vi "DHT11 Read (FPGA).vi"(0 "FPGA I/O In":refnum<k21>="ConnectorA/DIO0") -> (4 "Temperature (°C)":u8, 6 "Humidity (%)":u8, 15 "error out":errorcluster)   [LabVIEW 2015, in "DHT11 (FPGA).lvlib"]
doc: "Read Temperature and Humidity from DHT11 Sensor.\n\n\nError Codes\n========\n\nError -8001: Checksum Error\nError- 8002: Timeout Error"
uses:
  DHT11 (FPGA).lvlib
  Command.ctl
  <vilib>/Platform/TimedLoop/XDataNode/timing_clust.ctl
  <vilib>/Platform/TimedLoop/XDataNode/nitl_modes.ctl
  <vilib>/Platform/TimedLoop/XDataNode/wakeup.ctl
  <vilib>/rvi/Emulation/niFpgaSctlEmulationGetInTimedLoop.vi
  <vilib>/rvi/Emulation/niFpgaEmulationReportErrorSimple.vi
  <vilib>/rvi/Emulation/niFpgaGetClockAttributes.vi
  <vilib>/rvi/Emulation/niFpgaCriticalErrorInLSC.vi
  <vilib>/rvi/eio/common/nirviEmuTemplateMethod_errors.vi
  <vilib>/Platform/TimedLoop/XDataNode/XDataNode.xnode
  <vilib>/eio/EIOMethodNode/EIOMethodNode.xnode
  <vilib>/eio/EIONode/EIONode.xnode
  <vilib>/Platform/TimedLoop/XDataNode/XDNodeRunTimeDep.lvlib
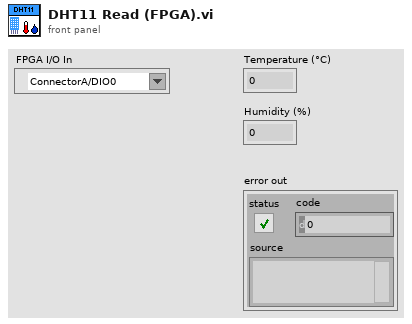
[diagram p1: front panel]
types:
  T1 = typedef "DHT11 (FPGA).lvlib/Command.ctl" = enum16{"Send Start Signal", "Wait Low", "Host Pulls Up", "Wait High", "Change to Read", "Wait for Sensor Response Signal Low", "Wait for Sensor Response Signal High", "Start Data Transmission", "Read Data", "Scale and Checksum", "Checksum Error", "Timeout Error"}
  T2 = typedef "XDNodeRunTimeDep.lvlib/timing_clust.ctl" = cluster{"Expected End [f-1]":u64, "Actual End [f-1]":u64, "Finished Late? [f-1]":bool, "Expected End [i-1]":u64, "Actual End [i-1]":u64, "Finished Late? [i-1]":bool, "Expected Start [i]":u64, "Actual Start [i]":u64, "Expected Start [f]":u64, "Actual Start [f]":u64, "Source Name":string, "Structure Name":string, "Period":i64, "Deadline":i64, "Offset":i64, "Start":i64, "Priority":i32, "Timeout":i32, "Mode":T3, "Wakeup Reason":T4, "Error":errorcluster, "Source Type":string, "Secondary Source Type":string, "Global End Time":u64, "Global Start Time":u64, "Frame Duration":u64, "Iteration Duration":u64, "Assigned CPU":i32, "I/O Scan Engine Mode":u32}
  T3 = typedef "XDNodeRunTimeDep.lvlib/nitl_modes.ctl" = enum32{"No Change", "Process missed periods, maintain original phase", "Discard missed periods, maintain original phase", "Process missed periods, ignore original phase", "Discard missed periods, ignore original phase"}
  T4 = typedef "XDNodeRunTimeDep.lvlib/wakeup.ctl" = enum32{"Normal", "Aborted", "Asynchronous wakeup", "Timing source error", "Timed loop error", "Timeout"}
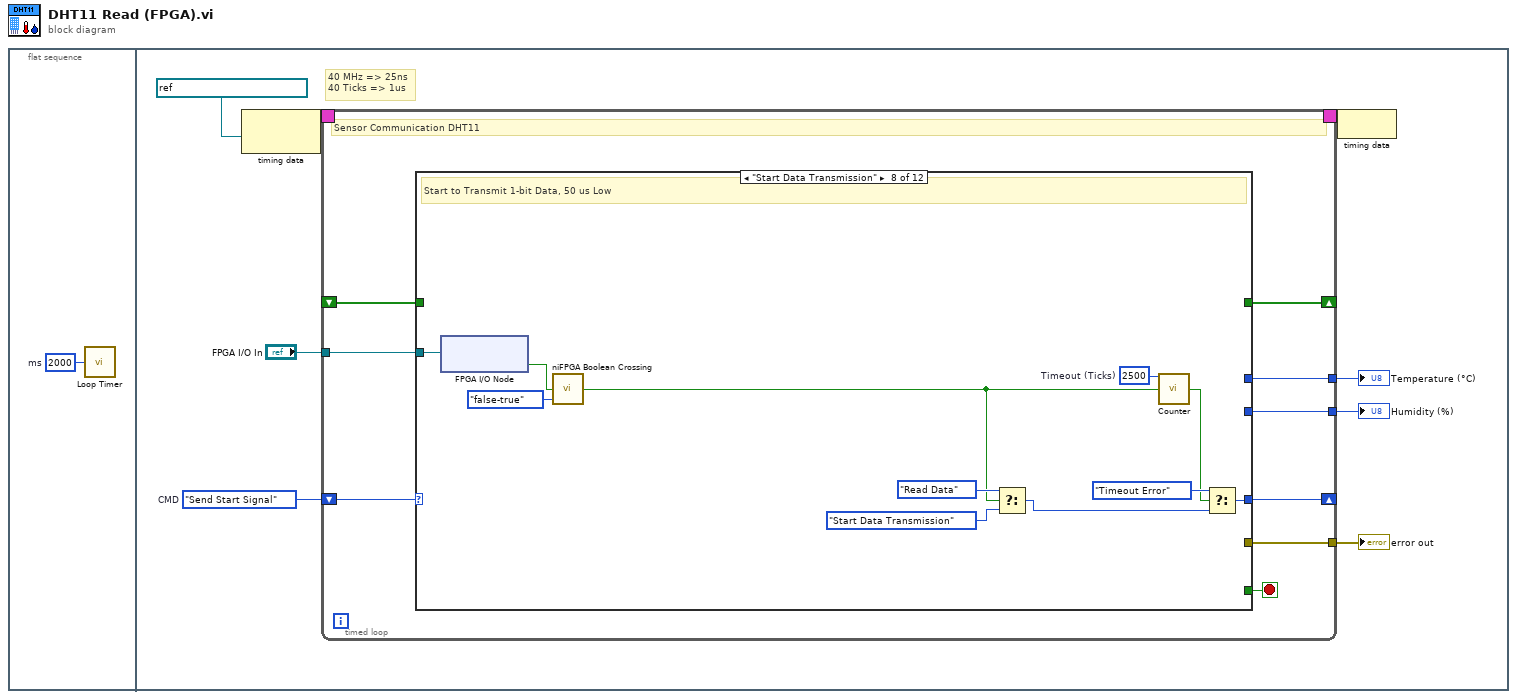
[diagram p0: block diagram]
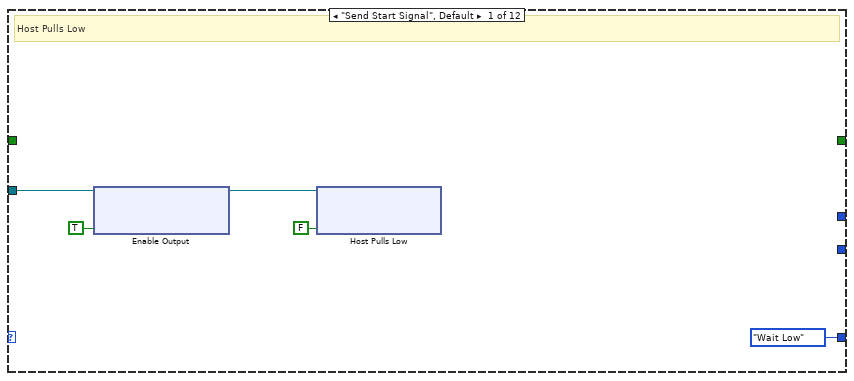
[diagram p2: hidden frame]
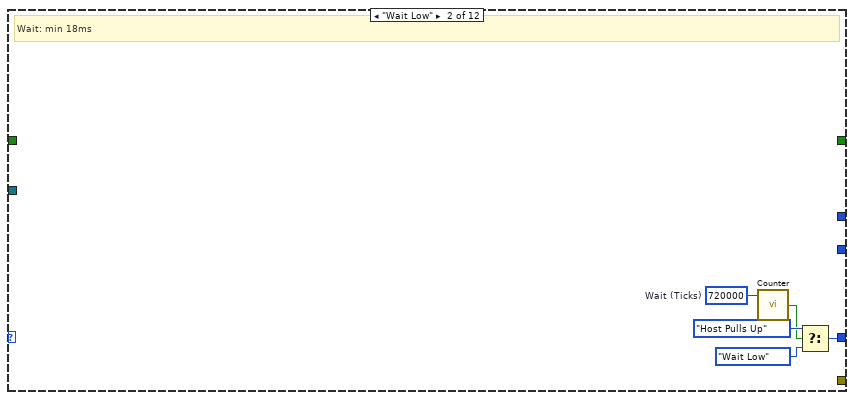
[diagram p3: hidden frame]
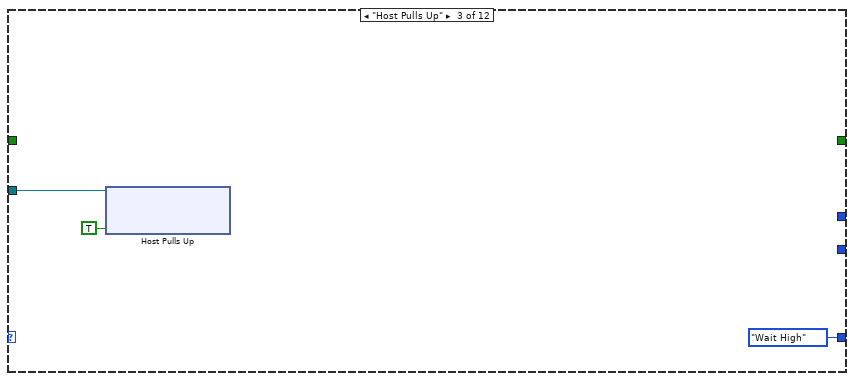
[diagram p4: hidden frame]
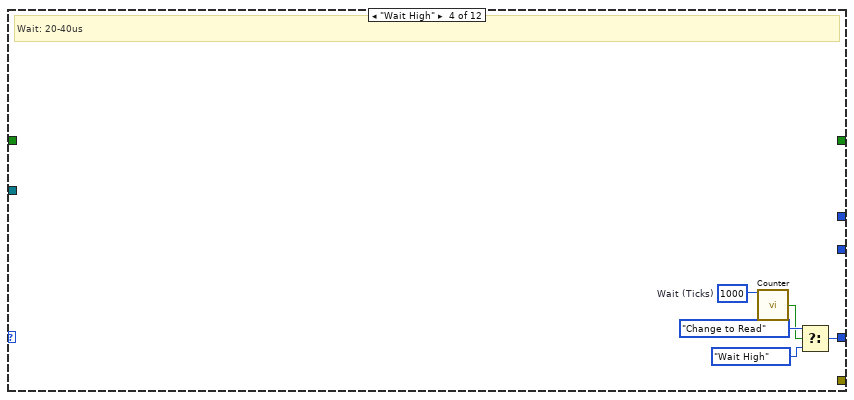
[diagram p5: hidden frame]
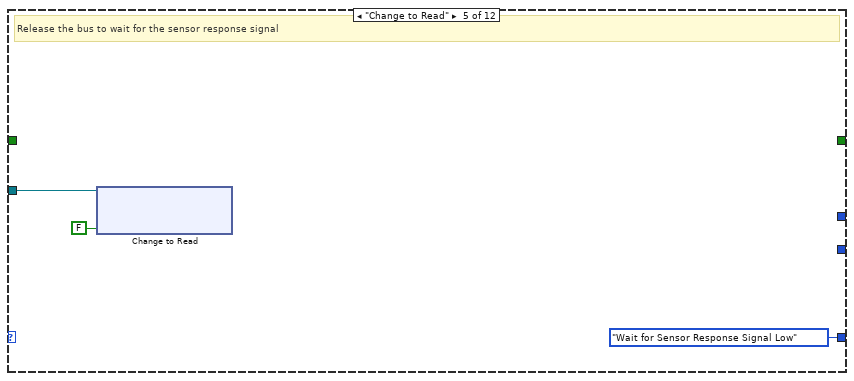
[diagram p6: hidden frame]
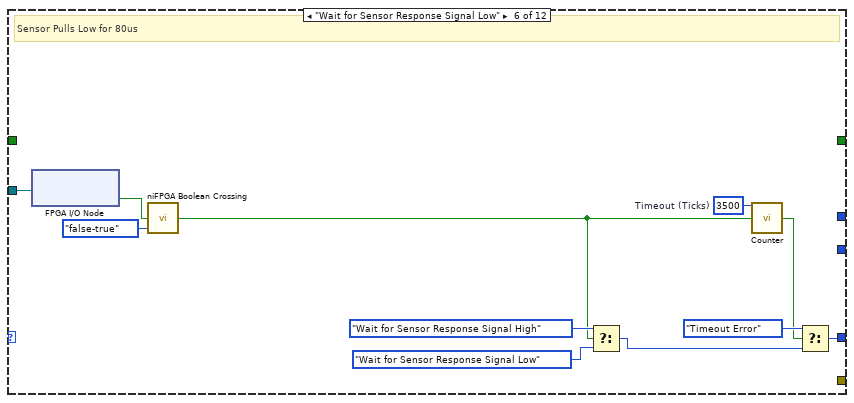
[diagram p7: hidden frame]
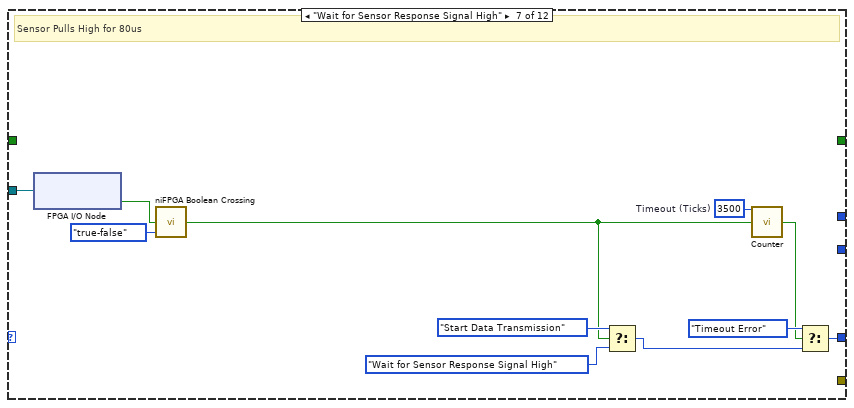
[diagram p8: hidden frame]
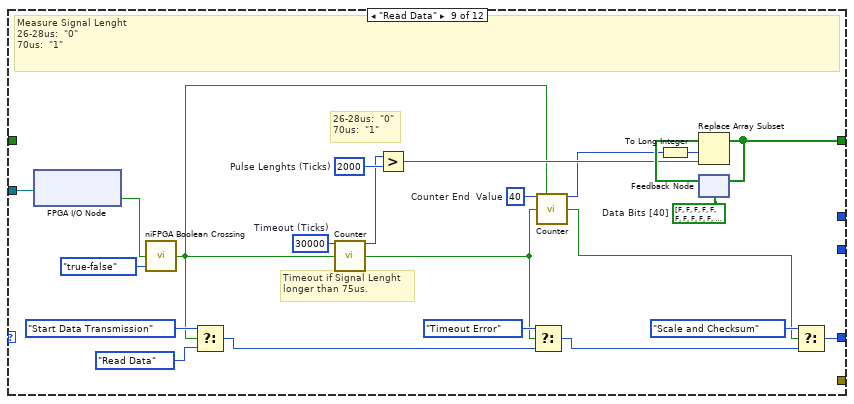
[diagram p9: hidden frame]
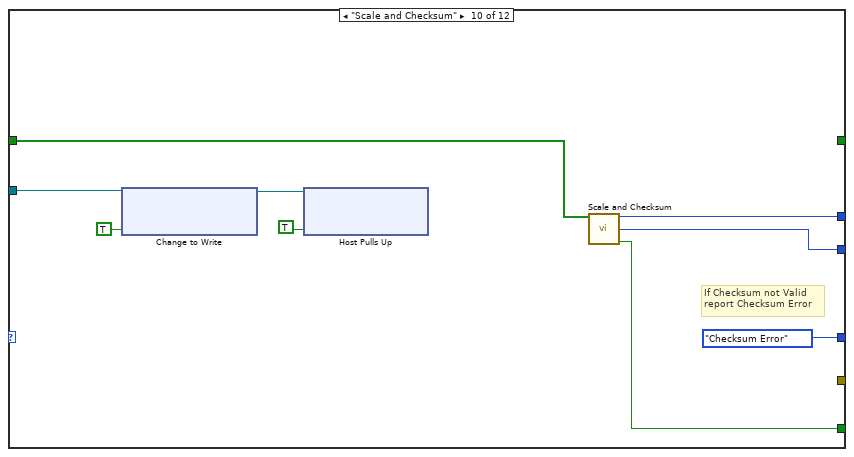
[diagram p10: hidden frame]
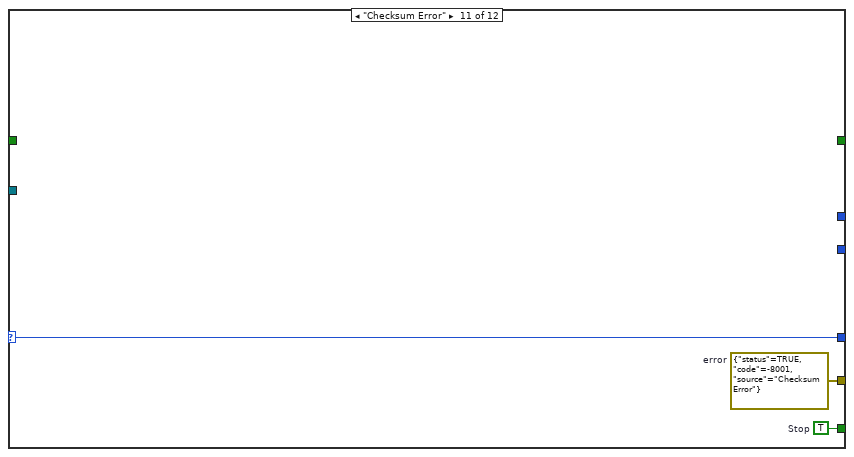
[diagram p11: hidden frame]
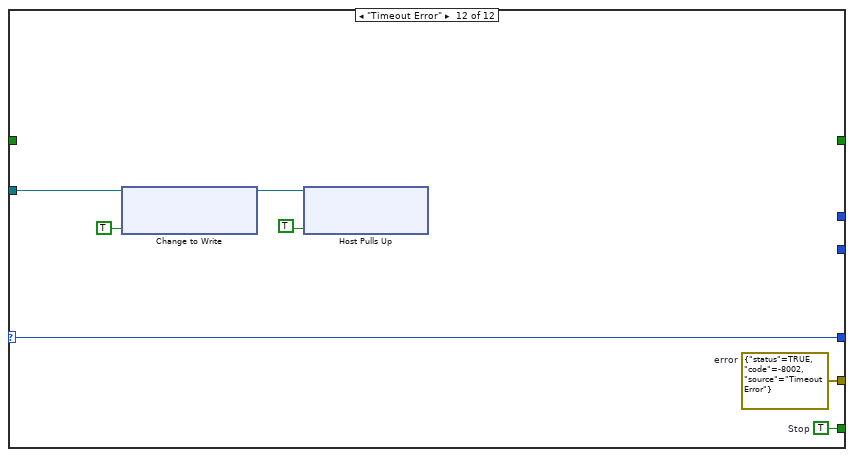
[diagram p12: hidden frame]
diagram:
  n1 = flat-sequence {
    frame #0 {
      w1 = u32 2000  # ms
      n2 = call "Loop Timer"("Count(mSec)"=w1) -> ()  [unwired: 1 out]
    }
    frame #1 {
      w7 = Command."Send Start Signal"  # CMD
      # "40 MHz => 25ns\n40 Ticks => 1us"
      n3 = node-c288(refnum<k21> "40 MHz Onboard Clock" ("Source Name")) -> (w9:T2)
      n4 = timed-loop {
        timing: w9 -> [_]
        timing-out: [_] -> w8
        shift-right: [w16] -> _
        shift-left: w7 -> [w18]
        tunnel: "FPGA I/O In" -> [w17]
        shift-right: [w14] -> _
        shift-left: _ -> [w13]
        tunnel: [w12] -> w5
        tunnel: [w11] -> w4
        tunnel: [w10] -> w3
        stop <- w15 stop-if-true
        # "Sensor Communication DHT11"
        n5 = case shown="\"Checksum Error\"" w18 {
          selector: w18 -> [_ _ _ _ _ _ _ _ _ _ w106 w113]
          tunnel: w17 -> [w22 _ w30 _ w38 w50 w61 w72 w95 w101 _ w109]
          tunnel: [Command."Wait Low" ("CMD") w26 Command."Wait High" ("CMD") w32 Command."Wait for Sensor Response Signal Low" ("CMD") w44 w55 w66 w76 Command."Checksum Error" ("CMD") w106 w113] -> w16
          tunnel: [_ _ _ _ _ _ _ _ _ w97 w107 w114] -> w15
          tunnel: [_ _ _ _ _ _ _ _ w74 _ _ _] -> w14
          tunnel: w13 -> [_ _ _ _ _ _ _ _ _ w100 _ _]
          tunnel: [_ _ _ _ _ _ _ _ _ w99 _ _] -> w12
          tunnel: [_ _ _ _ _ _ _ _ _ w98 _ _] -> w11
          tunnel: [_ _ _ _ _ _ _ _ _ _ w105 w108] -> w10
          frame "Send Start Signal", Default {
            # "Host Pulls Low"
            n6 = xnode "Enable Output"("FPGA I/O In"=w22, "Enable"=TRUE ("Data")) -> ("FPGA I/O Out"=w20:refnum<k21>)
            n7 = xnode "Host Pulls Low"("FPGA I/O In"=w20, "Data"=FALSE ("Enable")) -> ()  [unwired: 1 out]
          }
          frame "Wait Low" {
            w28 = u32 720000  # Wait (Ticks)
            # "Wait: min 18ms"
            n8 = call "Counter.vi"("Counter End  Value"=w28) -> ("End Reached"=w24:bool)  [unwired: 13 in, 1 out]
            n9 = Select(t=Command."Host Pulls Up" ("CMD"), s=w24, f=Command."Wait Low" ("CMD")) -> (s? t:f=w26:T1)
          }
          frame "Host Pulls Up" {
            n10 = xnode "Host Pulls Up"("FPGA I/O In"=w30, "Data"=TRUE ("Enable")) -> ()  [unwired: 1 out]
          }
          frame "Wait High" {
            w36 = u32 1000  # Wait (Ticks)
            # "Wait: 20-40us"
            n11 = call "Counter.vi"("Counter End  Value"=w36) -> ("End Reached"=w33:bool)  [unwired: 13 in, 1 out]
            n12 = Select(t=Command."Change to Read" ("CMD"), s=w33, f=Command."Wait High" ("CMD")) -> (s? t:f=w32:T1)
          }
          frame "Change to Read" {
            # "Release the bus to wait for the sensor response signal"
            n13 = xnode "Change to Read"("FPGA I/O In"=w38, "Enable"=FALSE ("Data")) -> ()  [unwired: 1 out]
          }
          frame "Wait for Sensor Response Signal Low" {
            w49 = u32 3500  # Timeout (Ticks)
            # "Sensor Pulls Low for 80us"
            n14 = xnode "FPGA I/O Node"("FPGA I/O In"=w50) -> ("I/O Item"=w45:bool)  [unwired: 1 out]
            n15 = call <vilib>:"niFPGA Boolean Crossing.vi"("input"=w45, "direction"=enum8{"either", "false-true", "true-false"}."false-true") -> ("crossing"=w40:bool)  [unwired: 7 in]
            n16 = Select(t=Command."Wait for Sensor Response Signal High" ("CMD"), s=w40, f=Command."Wait for Sensor Response Signal Low" ("CMD")) -> (s? t:f=w43:T1)
            n17 = call "Counter.vi"("Counter End  Value"=w49, "Reset"=w40) -> ("End Reached"=w41:bool)  [unwired: 12 in, 1 out]
            n18 = Select(t=Command."Timeout Error", s=w41, f=w43) -> (s? t:f=w44:T1)
          }
          frame "Wait for Sensor Response Signal High" {
            w60 = u32 3500  # Timeout (Ticks)
            # "Sensor Pulls High for 80us"
            n19 = xnode "FPGA I/O Node"("FPGA I/O In"=w61) -> ("I/O Item"=w56:bool)  [unwired: 1 out]
            n20 = call <vilib>:"niFPGA Boolean Crossing.vi"("input"=w56, "direction"=enum8{"either", "false-true", "true-false"}."true-false") -> ("crossing"=w51:bool)  [unwired: 7 in]
            n21 = Select(t=Command."Start Data Transmission" ("CMD"), s=w51, f=Command."Wait for Sensor Response Signal High" ("CMD")) -> (s? t:f=w54:T1)
            n22 = call "Counter.vi"("Counter End  Value"=w60, "Reset"=w51) -> ("End Reached"=w52:bool)  [unwired: 12 in, 1 out]
            n23 = Select(t=Command."Timeout Error", s=w52, f=w54) -> (s? t:f=w55:T1)
          }
          frame "Start Data Transmission" {
            w71 = u32 2500  # Timeout (Ticks)
            # "Start to Transmit 1-bit Data, 50 us Low"
            n24 = xnode "FPGA I/O Node"("FPGA I/O In"=w72) -> ("I/O Item"=w67:bool)  [unwired: 1 out]
            n25 = call <vilib>:"niFPGA Boolean Crossing.vi"("input"=w67, "direction"=enum8{"either", "false-true", "true-false"}."false-true") -> ("crossing"=w62:bool)  [unwired: 7 in]
            n26 = Select(t=Command."Read Data" ("CMD"), s=w62, f=Command."Start Data Transmission" ("CMD")) -> (s? t:f=w65:T1)
            n27 = call "Counter.vi"("Counter End  Value"=w71, "Reset"=w62) -> ("End Reached"=w63:bool)  [unwired: 12 in, 1 out]
            n28 = Select(t=Command."Timeout Error", s=w63, f=w65) -> (s? t:f=w66:T1)
          }
          frame "Read Data" {
            w94 = u32 30000  # Timeout (Ticks)
            w88 = u32 2000  # Pulse Lenghts (Ticks)
            w82 = u32 40  # Counter End  Value
            w86 = bool[] [FALSE, FALSE, FALSE, FALSE, FALSE, FALSE, FALSE, FALSE, FALSE, FALSE, FALSE, FALSE, FALSE, FALSE, FALSE, FALSE, FALSE, FALSE, FALSE, FALSE, FALSE, FALSE, FALSE, FALSE, FALSE, FALSE, FALSE, FALSE, FALSE, FALSE, FALSE, FALSE, FALSE, FALSE, FALSE, FALSE, FALSE, FALSE, FALSE, FALSE]  # Data Bits [40]
            # "26-28us:  \"0\"\n70us:  \"1\""
            # "Timeout if Signal Lenght\nlonger than 75us."
            # "Measure Signal Lenght\n26-28us:  \"0\"\n70us:  \"1\""
            n29 = xnode "FPGA I/O Node"("FPGA I/O In"=w95) -> ("I/O Item"=w90:bool)  [unwired: 1 out]
            n30 = call <vilib>:"niFPGA Boolean Crossing.vi"("input"=w90, "direction"=enum8{"either", "false-true", "true-false"}."true-false") -> ("crossing"=w79:bool)  [unwired: 7 in]
            n31 = Select(t=Command."Start Data Transmission" ("CMD"), s=w79, f=Command."Read Data" ("CMD")) -> (s? t:f=w78:T1)
            n32 = call "Counter.vi"("Counter End  Value"=w94, "Reset"=w79) -> ("Counter Value"=w87:u32, "End Reached"=w80:bool)  [unwired: 12 in]
            n33 = Greater?(x=w87, y=w88) -> (0:w83:bool)
            n34 = Select(t=Command."Timeout Error", s=w80, f=w78) -> (s? t:f=w75:T1)
            n35 = call "Counter.vi"("Counter End  Value"=w82, "Input Valid"=w79, "Reset"=w80) -> ("Counter Value"=w81:u32, "End Reached"=w73:bool)  [unwired: 11 in]
            n36 = To Long Integer(number=w81) -> (32bit integer=w84:i32)
            n37 = feedback #1(w86) -> (w85:bool[])
            n38 = Replace Array Subset(array=w85, new element=w83, index=w84) -> (w74:bool[])
            n39 = feedback-in #1(w74) -> ()
            n40 = Select(t=Command."Scale and Checksum", s=w73, f=w75) -> (s? t:f=w76:T1)
          }
          frame "Scale and Checksum" {
            # "If Checksum not Valid\nreport Checksum Error"
            n41 = xnode "Change to Write"("FPGA I/O In"=w101, "Enable"=TRUE ("Data")) -> ("FPGA I/O Out"=w102:refnum<k21>)
            n42 = xnode "Host Pulls Up"("FPGA I/O In"=w102, "Data"=TRUE ("Enable")) -> ()  [unwired: 1 out]
            n43 = call "Scale and Checksum.vi"("Raw Data"=w100) -> ("Temperature (°C)"=w99:u8, "Humidity (%)"=w98:u8, "Valid?"=w97:bool)  [unwired: 12 in]
          }
          frame "Checksum Error" {
            w105 = errorcluster {"status"=TRUE, "code"=-8001, "source"="Checksum Error"}  # error
            w107 = TRUE  # Stop
          }
          frame "Timeout Error" {
            w108 = errorcluster {"status"=TRUE, "code"=-8002, "source"="Timeout Error"}  # error
            w114 = TRUE  # Stop
            n44 = xnode "Change to Write"("FPGA I/O In"=w109, "Enable"=TRUE ("Data")) -> ("FPGA I/O Out"=w110:refnum<k21>)
            n45 = xnode "Host Pulls Up"("FPGA I/O In"=w110, "Data"=TRUE ("Enable")) -> ()  [unwired: 1 out]
          }
        }
      }
      "Temperature (°C)" <- w5
      "Humidity (%)" <- w4
      "error out" <- w3
      n46 = node-c288(w8) -> ()
    }
  }
